vi "Gasliste vergleichen.vi"(10 "FT-IR":bool) -> ()   [LabVIEW 2020, in "FT-IR.lvlib"]
uses:
  FT-IR.lvlib
  Visualisierungs Elemente/String - Ausgabefeld.ctl
  Visualisierungs Elemente/Button.ctl
  FGV FT-IR Gasliste Aktionen.ctl
  Sprachverwaltung/FGV Aktion Tabelle zerlegen.ctl
  EPA 1065/Allgemeine VIs/Aktion Wertaenderung Gasliste.ctl
  Messdaten/Aktionen FGV Messdaten.ctl
  Log Konfig/LogKonfig.lvlib
  Messdaten/Messdaten.lvlib
  Sprachverwaltung/Sprachverwaltung.lvlib
  EPA 1065/EPA 1065.lvlib
panel:
  in  "ABBRECHEN":T1
  in  "Übernehmen":T1
  out "Ausgelesene Gasliste":T2[](array[typedef])
  out "Aktuelle Gasliste":T2[](array[typedef])
  # "Vergleich Gaslisten"
  # "Aktuell verwendete Gasliste"
  # "Neue Gasliste"
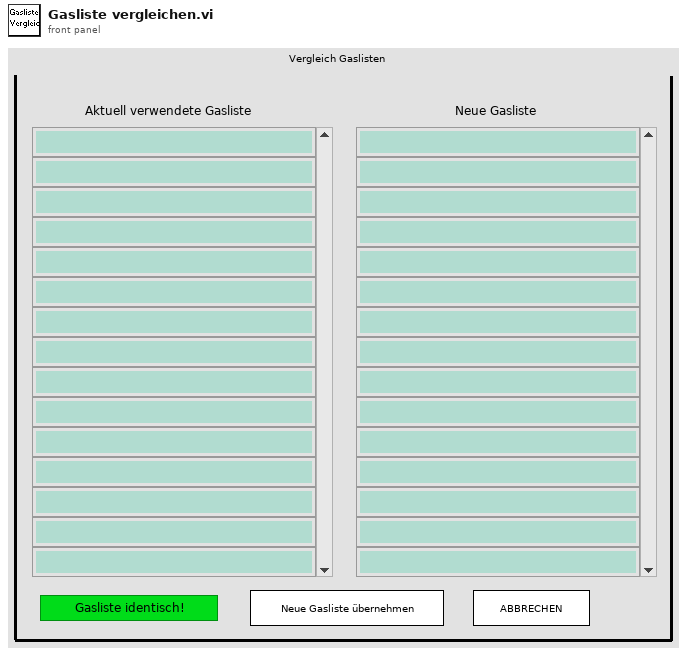
[diagram p1: front panel]
types:
  T1 = typedef "Button.ctl" = bool
  T2 = typedef "String - Ausgabefeld.ctl" = string
  T3 = typedef "Sprachverwaltung.lvlib/FGV Aktion Tabelle zerlegen.ctl" = enum16{"laden", "vereinzeln", "speichern"}
  T4 = enum8{"Enabled", "Disabled", "Disabled and Grayed Out"}
  T5 = typedef "FT-IR.lvlib/FGV FT-IR Gasliste Aktionen.ctl" = enum16{"lesen", "Gasliste FT-IR", "Gasliste ausgelesen", "laden", "speichern", "löschen"}
  T6 = typedef "EPA 1065.lvlib/Aktion Wertaenderung Gasliste.ctl" = enum16{"Init", "lesen", "Gasliste geändert", "ARN inaktiv", "LEAK inaktiv", "Interference 366 inaktiv", "T90 inaktiv", "Interference 375 inaktiv", "Chiller inaktiv", "FID O2 inaktiv", "FID Opti inaktiv", "Drift inaktiv", "Pre Test inaktiv", "LinV2 inaktiv"}
  T7 = typedef "Messdaten.lvlib/Aktionen FGV Messdaten.ctl" = enum16{"lesen", "schreiben", "löschen", "Mittelwerte", "Komponente"}
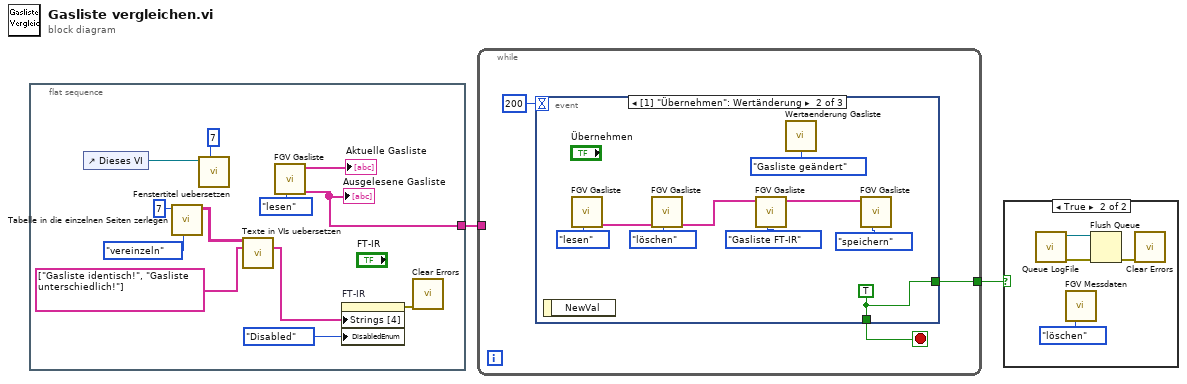
[diagram p0: block diagram]
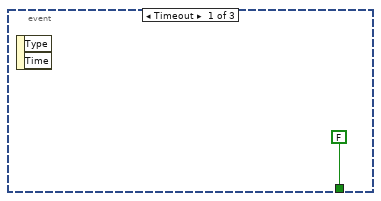
[diagram p3: hidden frame]
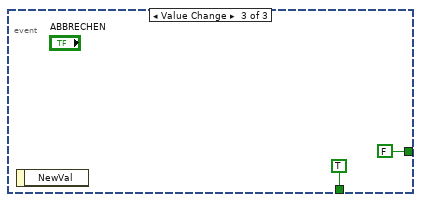
[diagram p4: hidden frame]
diagram:
  n1 = flat-sequence {
    tunnel: [w12] -> w2
    frame #0 {
      n2 = control-ref of="Dieses VI"() -> (w7:refnum<vi>)
      n3 = call "Tabelle in die einzelnen Seiten zerlegen.vi"("Aktion"=FGV_Aktion_Tabelle_zerlegen."vereinzeln", "Index (Seite)"=7) -> ("Sprachliste"=w4:string[][])  [unwired: 7 in, 2 out]
      n4 = call "Fenstertitel uebersetzen.vi"("Index (Seite)"=7, "Dieses VI"=w7) -> ()  [unwired: 6 in, 4 out]
      n5 = call "Texte in VIs uebersetzen.vi"("Sprachliste"=w4, "String-Array zum Übersetzen"=string[] ["Gasliste identisch!", "Gasliste unterschiedlich!"] ("Strings [4]")) -> ("String-Array zum Übersetzen"=w8:string[])  [unwired: 9 in, 4 out]
      n6 = call "FGV Gasliste.vi"("Aktionen"=FGV_FT-IR_Gasliste_Aktionen."lesen") -> ("Gasliste ausgelesen"=w12:T2[], "Aktuelle Gasliste FT-IR"=→"Aktuelle Gasliste":T2[])  [unwired: 8 in, 1 out]
      "Ausgelesene Gasliste" <- w12
      n7 = property on="FT-IR" class="Bool. (strikt)"("Strings [4]"=w8, "DisabledEnum"=T4."Disabled" ("Deaktiviert")) -> (error out=w10:errorcluster)  [unwired: 2 in, 1 out]
      n8 = call <vilib>:"Clear Errors.vi"("error in (no error)"=w10) -> ()  [unwired: 5 in, 2 out]
    }
  }
  n9 = while {
    tunnel: w2 -> [_]
    tunnel: [w15] -> w1
    stop <- w17 stop-if-true
    n10 = event shown="[1] \"Übernehmen\": Wertänderung" {
      selector: _ -> [_ _ _]
      dyn-events: _ -> [_ _ _]
      timeout: 200 -> [_ _ _]
      tunnel: [FALSE w23 TRUE] -> w17
      tunnel: [_ w23 FALSE] -> w15
      event Timeout {
        n11 = event-data() -> ()  [unwired: 1 in, 2 out]
      }
      event Value Change {
        w23 = TRUE
        n12 = event-data() -> ()  [unwired: 1 in, 1 out]
        n13 = call "FGV Gasliste.vi"("Aktionen"=FGV_FT-IR_Gasliste_Aktionen."lesen") -> ("Gasliste ausgelesen"=w21:T2[])  [unwired: 8 in, 2 out]
        n14 = call "FGV Gasliste.vi"("Aktionen"=FGV_FT-IR_Gasliste_Aktionen."löschen", "Gasliste ausgelesen"=w21) -> ("Gasliste ausgelesen"=w20:T2[])  [unwired: 7 in, 2 out]
        n15 = call "FGV Gasliste.vi"("Aktionen"=FGV_FT-IR_Gasliste_Aktionen."Gasliste FT-IR", "Aktuelle Gasliste FT-IR"=w20) -> ("Aktuelle Gasliste FT-IR"=w24:T2[])  [unwired: 7 in, 2 out]
        n16 = call "Wertaenderung Gasliste.vi"("Aktion"=Aktion_Wertaenderung_Gasliste."Gasliste geändert") -> ()  [unwired: 13 in, 2 out]
        n17 = call "FGV Gasliste.vi"("Aktionen"=FGV_FT-IR_Gasliste_Aktionen."speichern", "Aktuelle Gasliste FT-IR"=w24) -> ()  [unwired: 7 in, 3 out]
      }
      event Value Change {
        n18 = event-data() -> ()  [unwired: 1 in, 1 out]
      }
    }
  }
  n19 = case shown="True" w1 {
    frame False {
    }
    frame True {
      n20 = call "Queue LogFile.vi"() -> ("error out"=w33:errorcluster, "Queue (Ausgang)"=w32:refnum<queue>)  [unwired: 6 in]
      n21 = call "FGV Messdaten.vi"("Aktionen"=Aktionen_FGV_Messdaten."löschen") -> ()  [unwired: 6 in, 9 out]
      n22 = Flush Queue(queue=w32, error in (no error)=w33) -> (error out=w30:errorcluster)  [unwired: 2 out]
      n23 = call <vilib>:"Clear Errors.vi"("error in (no error)"=w30) -> ()  [unwired: 5 in, 2 out]
    }
  }
